vi "Config REM IO Mods.vi"(8 "error in (no error)":errorcluster, 10 "IOV Ref In":refnum<k21>, 11 "VS Ref In":T1=18446744073709551615 format="%.0x") -> (0 "error out":errorcluster, 2 "IOV Ref Out":refnum<k21>, 3 "VS Ref Out":T1=18446744073709551615 format="%.0x")   [LabVIEW 2019, in "Scan Engine Custom Device.lvlib"]
uses:
  Scan Engine Custom Device.lvlib
  <vilib>/NI VeriStand/Custom Device API/Custom Device Item Ref.ctl
  <vilib>/NI VeriStand/Custom Device API/Custom Device API.lvlib
  Modules.lvlibp/RemIO Module/RemIO Module.lvclass
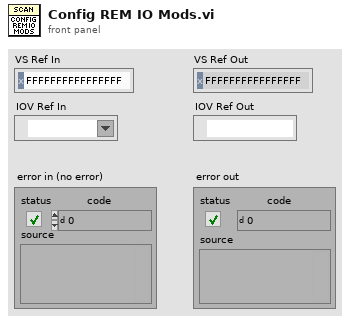
[diagram p1: front panel]
types:
  T1 = typedef "Custom Device API.lvlib/Custom Device Item Ref.ctl" = u64
  T2 = typedef "Modules.lvlibp/Custom Device API.lvlib/Custom Device Item Ref.ctl" = u64
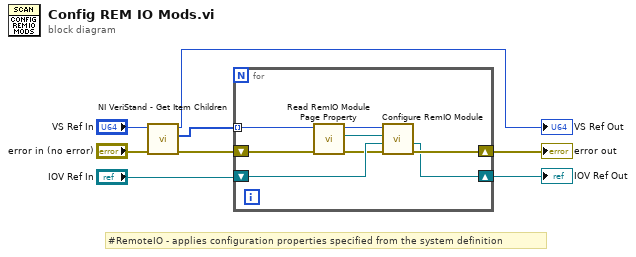
[diagram p0: block diagram]
diagram:
  # "#RemoteIO - applies configuration properties specified from the system definition"
  n1 = call <vilib>:"NI VeriStand - Get Item Children.vi"("error in (no error)"="error in (no error)", "Item Ref in"="VS Ref In") -> ("error out"=w2:errorcluster, "Child Refs"=w1:T1[], "Item Ref out"=→"VS Ref Out":T1)  [unwired: 6 in, 1 out]
  n2 = for {
    shift-right: [w14] -> w4
    shift-left: w2 -> [w16]
    shift-right: [w13] -> w5
    shift-left: "IOV Ref In" -> [w15]
    tunnel: w1 -> [w9] mode=indexing
    n3 = call "Read RemIO Module Page Property.vi"("error in (no error)"=w16, "Node Ptr In"=w9) -> ("error out"=w12:errorcluster, "RemIO Module"=w10:refnum<class "RemIO Module.lvclass">, "Node Ptr Out"=w11:T2)  [unwired: 7 in]
    n4 = call "Configure RemIO Module.vi"("error in (no error)"=w12, "Slave Ref In"=w15, "RemIO Module in"=w10, "Node Ptr In"=w11) -> ("error out"=w14:errorcluster, "Slave Ref Out"=w13:refnum<k21>)  [unwired: 4 in, 2 out]
  }
  "error out" <- w4
  "IOV Ref Out" <- w5
